vi "Read U64.vi"(8 "error in (no error)":errorcluster, 9 "Timeout (ms)":i32, 11 "CIFTag in":refnum<class "CIF_NIChn_U64.lvclass">) -> (0 "error out":errorcluster, 1 "timed out?":bool, 2 "Data":u64, 3 "CIFTag out":refnum<class "CIF_NIChn_U64.lvclass">)   [LabVIEW 2021, in "CIF_NIChn_U64.lvclass"]
uses:
  CIF_NIChn_U64.lvclass
  CIF_NIChn_U64.lvclass/CIF_NIChn_U64.ctl
  CIFChannels/Typedef/Direction.ctl
  CIFChannels/CIFChannels.lvclass
  CIFChannels/Typedef/Channel State.ctl
  NIChn/CIF_NIChn.lvclass
  cbead010-ab61-49ec-ac6c-083511305d37.vi
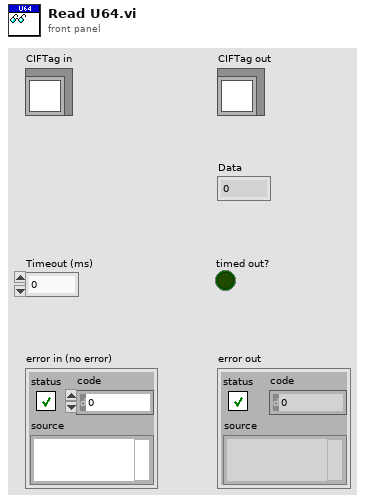
[diagram p1: front panel]
types:
  T1 = typedef "CIFChannels.lvclass/Channel State.ctl" = enum16{"Creating", "Disconnected", "Connecting", "Connected", "Destroyed"}
  T2 = typedef "CIFChannels.lvclass/Direction.ctl" = enum16{"Publisher", "Subscriber"}
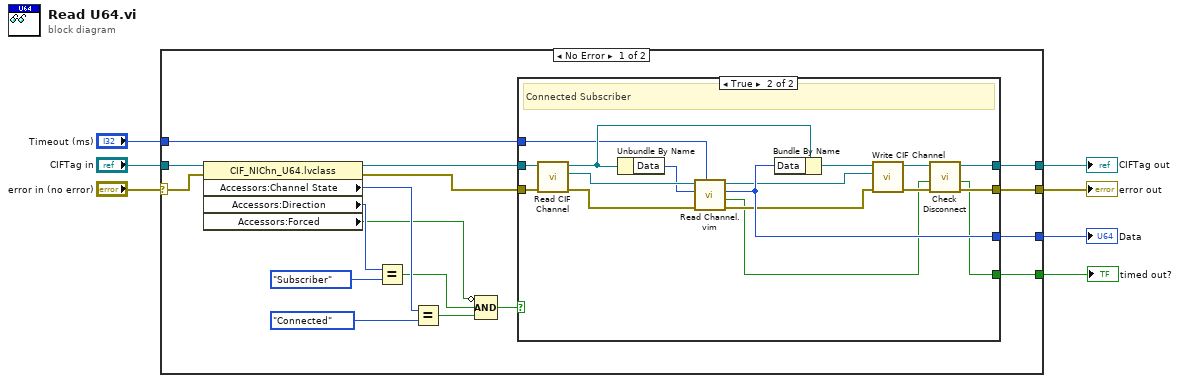
[diagram p0: block diagram]
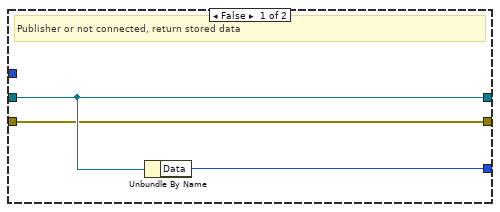
[diagram p2: hidden frame]
diagram:
  n1 = case shown="No Error" "error in (no error)" {
    selector: "error in (no error)" -> [w21 w46]
    tunnel: [w10 w46] -> w6
    tunnel: [w11 w45] -> w4
    tunnel: "CIFTag in" -> [w22 w45]
    tunnel: [w24 _] -> w3
    tunnel: [w23 _] -> w2
    tunnel: "Timeout (ms)" -> [w9 _]
    frame No Error {
      n2 = property class="CIF_NIChn_U64.lvclass"(reference=w22, error in=w21) -> (reference out=w20:refnum<class "CIF_NIChn_U64.lvclass">, error out=w19:errorcluster, "Accessors:Channel State"=w16:T1, "Accessors:Direction"=w18:T2, "Accessors:Forced"=w8:bool)
      n3 = Equal?(x=w18, y=Direction."Subscriber") -> (x = y?=w12:bool)
      n4 = Equal?(x=w16, y=Channel_State."Connected") -> (x = y?=w14:bool)
      n5 = Compound Arithmetic op=AND(invert w8, w12, w14) -> (w13:bool)
      n6 = case shown="True" w13 {
        tunnel: [_ w30] -> w24
        tunnel: [w27 w37] -> w23
        tunnel: w19 -> [w25 w43]
        tunnel: w20 -> [w26 w44]
        tunnel: [w26 w42] -> w11
        tunnel: [w25 w41] -> w10
        tunnel: w9 -> [_ w29]
        frame False {
          # "Publisher or not connected, return stored data"
          n7 = Unbundle By Name(w26) -> ("Data"=w27:u64)
        }
        frame True {
          # "Connected Subscriber"
          n8 = call "Read CIF Channel.vi"("error in (no error)"=w43, "CIFTag in"=w44) -> ("error out"=w38:errorcluster, "CIF Channel"=w39:refnum<k21>, "CIFTag out"=w40:refnum<class "CIF_NIChn_U64.lvclass">)  [unwired: 7 in]
          n9 = Unbundle By Name(w40) -> ("Data"=w28:u64)
          n10 = call "Read Channel.vim"("Timeout (ms)"=w29, "error in"=w38, "Data in"=w28, "CIF Channel in"=w39) -> ("error out"=w35:errorcluster, "Timed out?"=w31:bool, "Data out"=w37:u64, "CIF Channel out"=w34:refnum<k21>)  [unwired: 4 in]
          n11 = Bundle By Name(cluster=w40, "Data"=w37) -> (w36:refnum<class "CIF_NIChn_U64.lvclass">)
          n12 = call "Write CIF Channel.vi"("error in (no error)"=w35, "CIF Channel"=w34, "CIFTag in"=w36) -> ("error out"=w32:errorcluster, "CIFTag out"=w33:refnum<class "CIF_NIChn_U64.lvclass">)  [unwired: 7 in]
          n13 = call "Check Disconnect.vi"("error in (no error)"=w32, "timeout in"=w31, "CIFTag in"=w33) -> ("error out"=w41:errorcluster, "timeout out"=w30:bool, "CIFTag out"=w42:refnum<class "CIF_NIChn_U64.lvclass">)  [unwired: 5 in, 1 out]
        }
      }
    }
    frame Error {
    }
  }
  "error out" <- w6
  "CIFTag out" <- w4
  "timed out?" <- w3
  "Data" <- w2
